vi "UE9 Externally Triggered Stream Example.vi"() -> ()   [LabVIEW 2021]
panel:
  in  "FirstFound":bool=TRUE
  in  "ConnectionType":u16(ring) items=["LJ_ctUSB", "LJ_ctETHERNET"]
  in  "Address":string="192.168.1.209"
  in  "AIN Range":u16(ring) items=["LJ_rgBIP5V", "LJ_rgUNI5V", "LJ_rgUNI2P5V", "LJ_rgUNI1P25V", "LJ_rgUNIP625V"]
  out "ms Per Loop":u32
  out "Comm Backlog":i32
  out "# Scans Read":i32
  out "# of iterations":i32
  out "Data":dbl[][](array[numeric]) format="%.3f"
  in  "Scan List":u8[](array[numeric])=[0, 1, 193, 194, 200, 224, 210, 224]
  in  "stop":bool
  out "Error Message":string
  in  "Resolution":i32=12
  # "Demonstrates an externally triggered stream on a single UE9.\n\nFIO0 = Timer0 (SystemTimerLow:  Can be used as a timestamp for each scan).\nFIO1 = Timer1 (FreqOut:  5000 Hz square wave can be used as trigger signal).\nFIO2 = Counter0\nFIO3 = External Trigger Input (Counter1)\n\nConnect the external trigger signal to FIO3, or connect FIO1 to FIO3 to provide a 5 kHz trigger.  Each falling edge on the trigger input\nwill cause a scan to occur, but realize that it takes at least 16 samples (or 64 samples for USB) before a packet of data is transferred from\nthe UE9 to the host.  You will not be able to manually tap a ground wire on FIO3 to create pulses.  The bouncing will cause some pulses\nto be too close together and cause an error.  Instead good clean pulses are required, and a new pulse cannot occur before the previous\nscan is completed.\n\nTested with UD V2.73, Comm firmware V1.40, and Control firmware V1.77."
  # "AIN0"
  # "AIN1"
  # "EIO_FIO0"
  # "MIO_CIO"
  # "Specify an IP address for Ethernet, or Local ID\nfor USB.  If FirstFound is selected, Local ID is\nignored for USB.  Clear FirstFound if using Ethernet."
  # "Timer0 LSW"
  # "Timer0 MSW"
  # "Counter0 LSW"
  # "(for all channels)"
  # "Counter0 MSW"
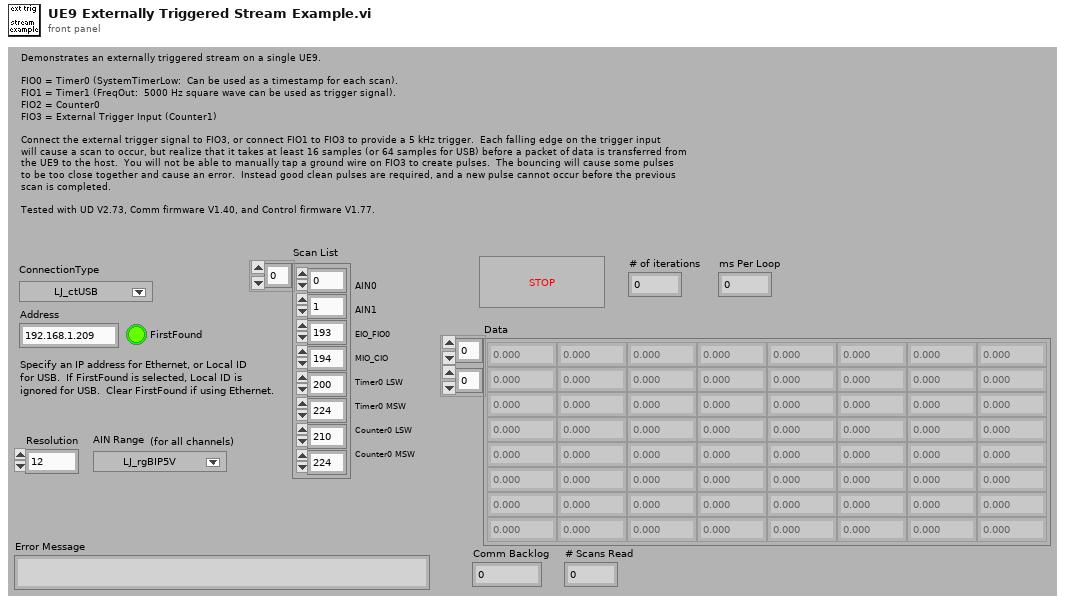
[diagram p1: front panel]
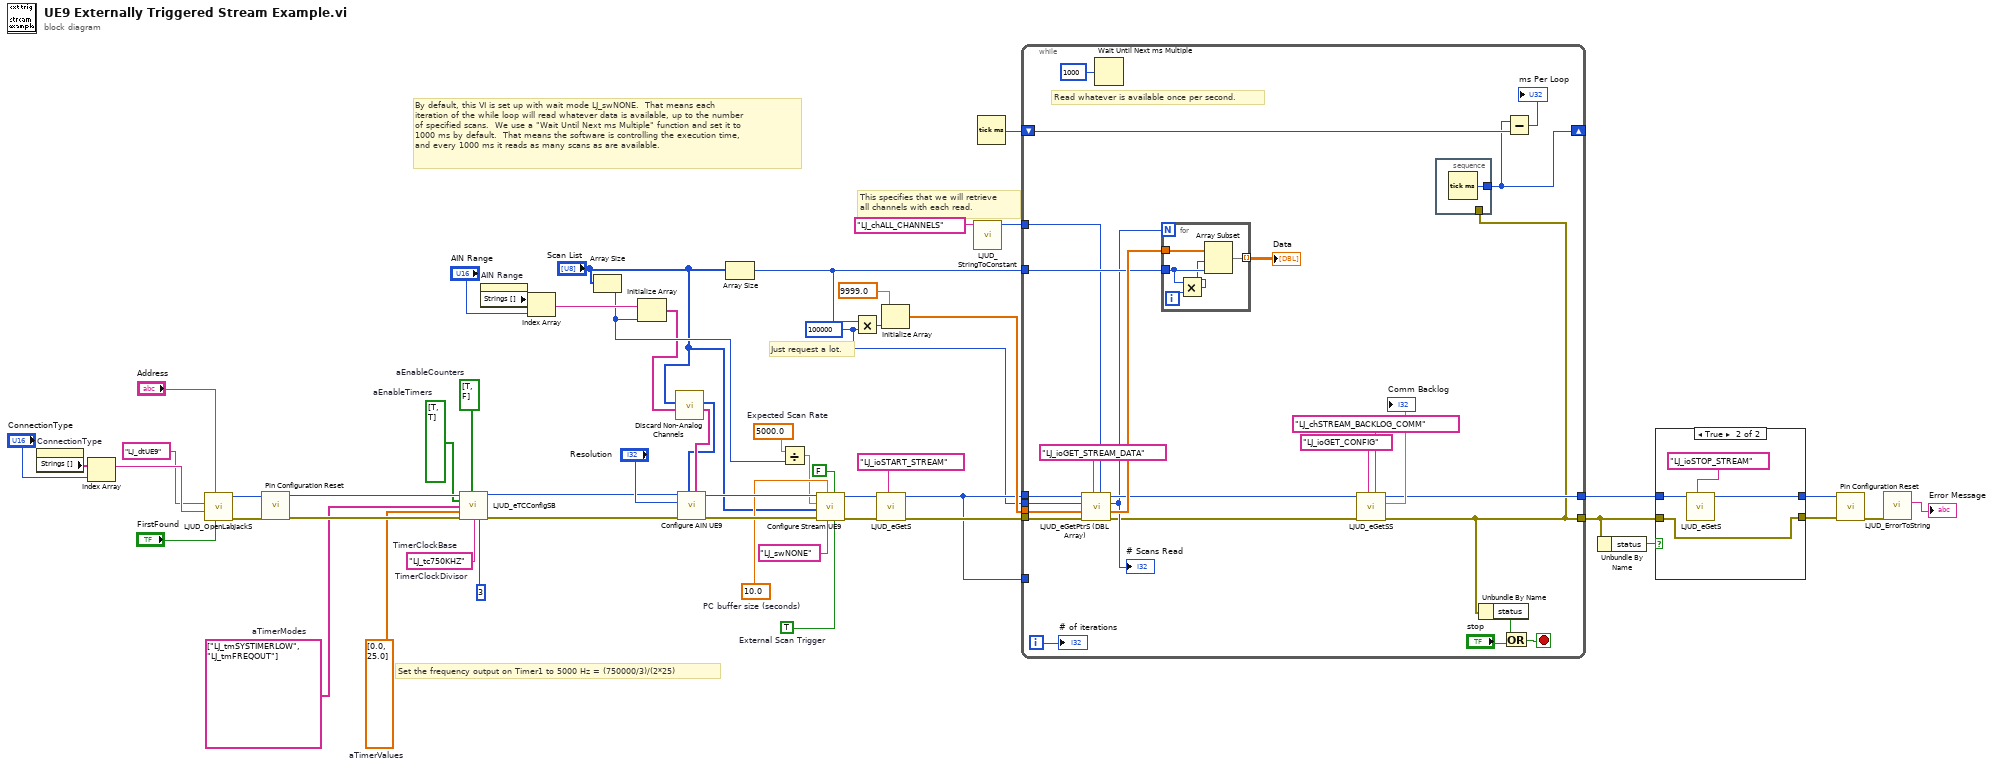
[diagram p0: block diagram]
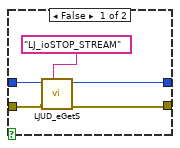
[diagram p2: hidden frame]
diagram:
  w4 = 3  # TimerClockDivisor
  w5 = "LJ_tc750KHZ"  # TimerClockBase
  w6 = dbl[] [0.0, 25.0]  # aTimerValues
  w7 = string[] ["LJ_tmSYSTIMERLOW", "LJ_tmFREQOUT"]  # aTimerModes
  w8 = bool[] [TRUE, TRUE]  # aEnableTimers
  w9 = bool[] [TRUE, FALSE]  # aEnableCounters
  w22 = 100000 ("y")
  w23 = TRUE  # External Scan Trigger
  w26 = 5000.0  # Expected Scan Rate
  w36 = 10.0  # PC buffer size (seconds)
  # "Set the frequency output on Timer1 to 5000 Hz = (750000/3)/(2*25)"
  # "This specifies that we will retrieve\nall channels with each read."
  # "Just request a lot."
  # "By default, this VI is set up with wait mode LJ_swNONE.  That means each\niteration of the while loop will read whatever data is available, up to the number\nof specified scans.  We use a \"Wait Until Next ms Multiple\" function and set it to\n1000 ms by default.  That means the software is controlling the execution time,\nand every 1000 ms it reads as many scans as are available."
  n1 = property on="ConnectionType" class="Ring (strict)"() -> ("Strings []"=w31:string[])  [unwired: 2 in, 2 out]
  n2 = Index Array(array=w31, index="ConnectionType") -> (element=w38:string)
  n3 = call "LJUD_OpenLabJackS.vi"("FirstFound"="FirstFound", "Address"="Address", "ConnectionType"=w38, "DeviceType"="LJ_dtUE9") -> ("error out"=w13:errorcluster, "Handle"=w11:i32)  [unwired: 5 in, 1 out]
  n4 = call "Pin Configuration Reset.vi"("error in"=w13, "Handle In"=w11) -> ("error out"=w12:errorcluster, "Handle Out"=w10:i32)  [unwired: 8 in]
  n5 = call "LJUD_eTCConfigSB.vi"("Handle In"=w10, "aEnableCounters"=w9, "aEnableTimers"=w8, "aTimerModes"=w7, "aTimerValues"=w6, "error in"=w12, "TimerClockBase"=w5, "TimerClockDivisor"=w4) -> ("Handle Out"=w2:i32, "error out"=w3:errorcluster)  [unwired: 6 in]
  n6 = property on="AIN Range" class="Ring (strict)"() -> ("Strings []"=w43:string[])  [unwired: 2 in, 2 out]
  n7 = Index Array(array=w43, index="AIN Range") -> (element=w41:string)
  n8 = Array Size(array="Scan List") -> (size(s)=w25:i32)
  n9 = Initialize Array(w41, w25) -> (w18:string[])
  n10 = call "Discard Non-Analog Channels.vi"("Ranges In"=w18, "Channels In"="Scan List") -> ("Ranges Out"=w17:string[], "Channels Out"=w16:i32[])  [unwired: 6 in, 2 out]
  n11 = call "Configure AIN UE9.vi"("Ranges"=w17, "Channels"=w16, "error in"=w3, "Resolution"="Resolution", "Handle In"=w2) -> ("error out"=w49:errorcluster, "Handle Out"=w47:i32)  [unwired: 5 in]
  n12 = Array Size(array="Scan List") -> (size(s)=w52:i32)
  n13 = Divide(x=w26, y=w25) -> (x/y=w24:dbl)
  n14 = call "Configure Stream UE9.vi"("External Scan Trigger"=w23, "Scan Clock Output"=FALSE ("External Scan Trigger"), "Wait Mode"="LJ_swNONE", "PC buffer size (seconds)"=w36, "error in"=w49, "Scan List"="Scan List", "Scan Rate (Hz)"=w24, "Handle In"=w47) -> ("error out"=w48:errorcluster, "Handle Out"=w46:i32)  [unwired: 1 in, 1 out]
  n15 = Multiply(x=w52, y=w22) -> (x*y=w55:i32)
  n16 = call "LJUD_eGetS.vi"("IOType"="LJ_ioSTART_STREAM", "error in"=w48, "Handle In"=w46) -> ("error out"=w33:errorcluster, "Handle Out"=w32:i32)  [unwired: 6 in, 1 out]
  n17 = Initialize Array(9999.0, w55) -> (w53:dbl[])
  n18 = call "LJUD_StringToConstant.vi"("String"="LJ_chALL_CHANNELS") -> ("Constant Number"=w20:i32)  [unwired: 9 in, 1 out]
  n19 = Tick Count (ms)() -> (millisecond timer value=w50:u32)
  n20 = while {
    tunnel: w20 -> [w56]
    tunnel: w22 -> [w57]
    tunnel: [w65] -> w44
    tunnel: w32 -> [_]
    shift-left: w50 -> [w73]
    shift-right: [w72] -> _
    tunnel: [w58] -> w40
    tunnel: w52 -> [w62]
    tunnel: w53 -> [w64]
    tunnel: w33 -> [w77]
    tunnel: w32 -> [w78]
    i -> [w74]
    stop <- w69 stop-if-true
    # "Read whatever is available once per second."
    n21 = call "LJUD_eGetPtrS (DBL Array).vi"("Channel"=w56, "IOType"="LJ_ioGET_STREAM_DATA", "error in"=w77, "DBL Array Write"=w64, "Value"=w57, "Handle In"=w78) -> ("error out"=w59:errorcluster, "DBL Array Read"=w76:dbl[], "Value"=w61:i32, "Handle Out"=w66:i32)  [unwired: 2 in]
    "# Scans Read" <- w61
    n22 = Wait Until Next ms Multiple(millisecond multiple=u32 1000) -> ()  [unwired: 1 out]
    n23 = for {
      N: w61 -> [_]
      tunnel: w76 -> [w86]
      tunnel: w62 -> [w85]
      tunnel: [w82] -> w75 mode=indexing
      i -> [w84]
      n24 = Multiply(x=w85, y=w84) -> (x*y=w83:i32)
      n25 = Array Subset(array=w86, index=w83, length=w85) -> (w82:dbl[])
    }
    "Data" <- w75
    n26 = call "LJUD_eGetSS.vi"("Channel"="LJ_chSTREAM_BACKLOG_COMM", "IOType"="LJ_ioGET_CONFIG", "error in"=w59, "Handle In"=w66) -> ("error out"=w58:errorcluster, "Value Read"=→"Comm Backlog":dbl, "Handle Out"=w65:i32)  [unwired: 5 in]
    n27 = stacked-sequence {
      tunnel: [w81] -> w72
      tunnel: w58 -> [_]
      frame #0 {
        n28 = Tick Count (ms)() -> (millisecond timer value=w81:u32)
      }
    }
    n29 = Unbundle By Name(w58) -> ("status"=w79:bool)
    n30 = Or(x=w79, y="stop") -> (x .or. y?=w69:bool)
    n31 = Subtract(x=w72, y=w73) -> (x-y=→"ms Per Loop":u32)
    "# of iterations" <- w74
  }
  n32 = Unbundle By Name(w40) -> ("status"=w39:bool)
  n33 = case shown="True" w39 {
    tunnel: [w88 w92] -> w15
    tunnel: w44 -> [w90 w94]
    tunnel: w40 -> [w89 w92]
    tunnel: [w87 w93] -> w1
    frame False {
      n34 = call "LJUD_eGetS.vi"("IOType"="LJ_ioSTOP_STREAM", "error in"=w89, "Handle In"=w90) -> ("error out"=w88:errorcluster, "Handle Out"=w87:i32)  [unwired: 6 in, 1 out]
    }
    frame True {
      n35 = call "LJUD_eGetS.vi"("IOType"="LJ_ioSTOP_STREAM", "Handle In"=w94) -> ("Handle Out"=w93:i32)  [unwired: 7 in, 2 out]
    }
  }
  n36 = call "Pin Configuration Reset.vi"("error in"=w15, "Handle In"=w1) -> ("error out"=w14:errorcluster)  [unwired: 8 in, 1 out]
  n37 = call "LJUD_ErrorToString.vi"("error in"=w14) -> ("String"=→"Error Message":string)  [unwired: 10 in]
